vi "OAT AC DC Separation.vi"   [LabVIEW 2017, in "SoundVib_OAUtility.lvlib"]
doc: "Separates and returns the AC and DC levels of the <B>even-angle signal</B> by continuously removing the DC values from the signal. This VI calculates the DC values over the interval specified by the <B>revolution number</B>. Wire data to the <B>even-angle signal</B> input to determine the polymorphic instance to use or manually select the instance."
uses:
  <vilib>/addons/Sound and Vibration/Order Analysis/Utility/SoundVib_OAUtility.lvlib
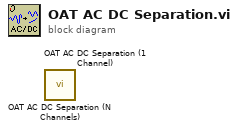
[diagram p0: block diagram]
diagram:
  n1 = call <vilib>:"OAT AC DC Separation (N Channels).vi"() -> ()  [unwired: 14 in, 6 out]
  n2 = call <vilib>:"OAT AC DC Separation (1 Channel).vi"() -> ()  [unwired: 14 in, 6 out]
